vi "Potting Data from Inspect Modules.vi"() -> ()   [LabVIEW 2011]
uses:
  Procedure Classes/Potting Procedure/Type Definitions/Inspect Modules - Module.ctl
  Shared Components/Vec3d Class/Vec3d Class.lvclass
  Shared Components/Utils/Type Definitions/Multi-Fiducial Image.ctl
  Shared Components/Utils/Type Definitions/Physical Image.ctl
  <vilib>/vision/Image Controls.llb/IMAQ Image.ctl
  Shared Components/Utils/Type Definitions/Fiducial with Source.ctl
  Shared Components/Utils/Type Definitions/Fiducial Image.ctl
  Shared Components/SyringeTool Class/Type Definitions/Module Potting Data.ctl
  Shared Components/Utils/Type Definitions/3d Line.ctl
  Shared Components/Utils/Type Definitions/3d Point.ctl
panel:
  out "Module Potting Data":T1
  out "error out":errorcluster
  in  "error in":errorcluster
  in  "Module Data":T4={"TBM-TBM"={"Fiducial Image"={"Image Position"=refnum, "Image Reference"=refnum, "Field of View"={"x(mm)"=0.0, "y(mm)"=0.0}}, "Fiducials"=[]}, "TBM-HDI"={"Fiducial Image"={"Image Position"=refnum, "Image Reference"=refnum, "Field of View"={"x(mm)"=0.0, "y(mm)"=0.0}}, "Fiducials"=[]}, "Address Pads"={"Fiducial Image"={"Image Position"=refnum, "Image Reference"=refnum, "Field of View"={"x(mm)"=0.0, "y(mm)"=0.0}}, "Fiducials"=[]}, "HDI Bond Pad References"=[], "BBM Bond Pad References"=[], "HV-HDI"={"Fiducial Image"={"Image Position"=refnum, "Image Reference"=refnum, "Field of View"={"x(mm)"=0.0, "y(mm)"=0.0}}, "Selected Fiducial"={"Fiducial Image Coordinate"=refnum, "Fiducial Source"=enum."Pattern Recognition"}, "fiducial name"=""}, "HV-BBM"={"Fiducial Image"={"Image Position"=refnum, "Image Reference"=refnum, "Field of View"={"x(mm)"=0.0, "y(mm)"=0.0}}, "Selected Fiducial"={"Fiducial Image Coordinate"=refnum, "Fiducial Source"=enum."Pattern Recognition"}, "fiducial name"=""}, "Chuck"=0, "Slot"=0, "Potting Selection"={"HDI Bond Pads"=[TRUE, TRUE, TRUE, TRUE, TRUE, TRUE, TRUE, TRUE, TRUE, TRUE, TRUE, TRUE, TRUE, TRUE, TRUE, TRUE], "BBM Bond Pads"=[TRUE, TRUE, TRUE, TRUE, TRUE, TRUE, TRUE, TRUE, TRUE, TRUE, TRUE, TRUE, TRUE, TRUE, TRUE, TRUE], "TBM Inner"={"Top"=TRUE, "Left"=TRUE, "Bottom"=TRUE, "Right"=TRUE}, "TBM Outer"={"Top"=TRUE, "Left"=TRUE, "Bottom"=TRUE, "Right"=TRUE}, "Address Pads"={"Top"=TRUE, "Bottom"=TRUE}, "High Voltage"={"HDI"=TRUE, "BBM"=TRUE}}}
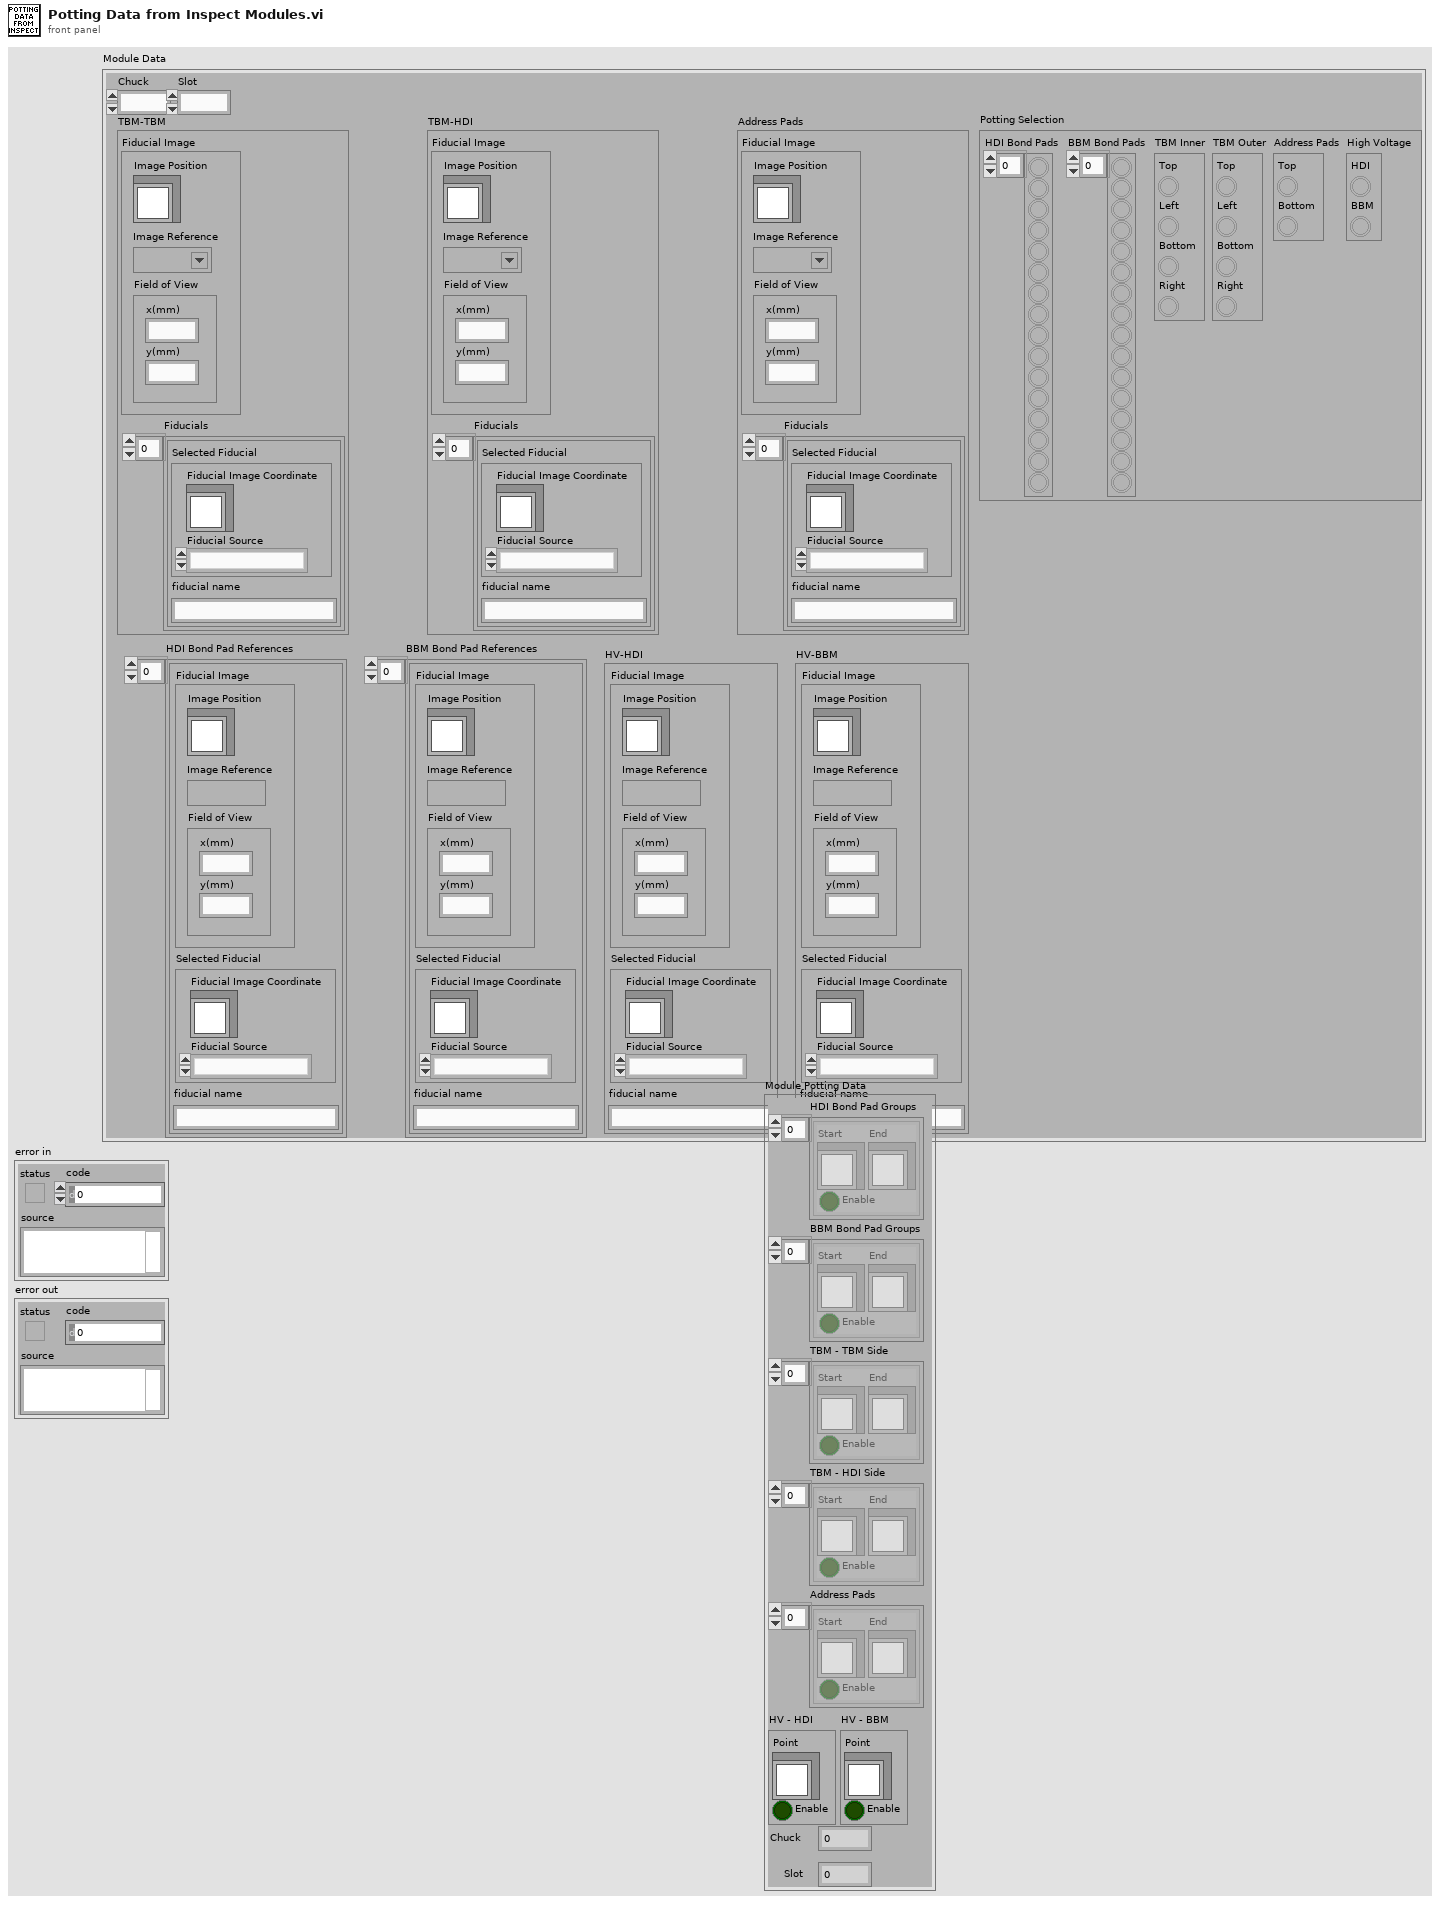
[diagram p1: front panel]
types:
  T1 = typedef "Module Potting Data.ctl" = cluster{"HDI Bond Pad Groups":T2[], "BBM Bond Pad Groups":T2[], "TBM - TBM Side":T2[], "TBM - HDI Side":T2[], "Address Pads":T2[], "Chuck":i32, "Slot":i32, "HV - HDI":T3, "HV - BBM":T3}
  T2 = typedef "3d Line.ctl" = cluster{"Start":refnum<class "Vec3d Class.lvclass">, "End":refnum<class "Vec3d Class.lvclass">, "Enable":bool}
  T3 = typedef "3d Point.ctl" = cluster{"Point":refnum<class "Vec3d Class.lvclass">, "Enable":bool}
  T4 = typedef "Inspect Modules - Module.ctl" = cluster{"TBM-TBM":T5, "TBM-HDI":T5, "Address Pads":T5, "HDI Bond Pad References":T9[], "BBM Bond Pad References":T9[], "HV-HDI":T9, "HV-BBM":T9, "Chuck":i32, "Slot":i32, "Potting Selection":cluster{"HDI Bond Pads":bool[], "BBM Bond Pads":bool[], "TBM Inner":cluster{"Top":bool, "Left":bool, "Bottom":bool, "Right":bool}, "TBM Outer":cluster{"Top":bool, "Left":bool, "Bottom":bool, "Right":bool}, "Address Pads":cluster{"Top":bool, "Bottom":bool}, "High Voltage":cluster{"HDI":bool, "BBM":bool}}}
  T5 = typedef "Multi-Fiducial Image.ctl" = cluster{"Fiducial Image":T6, "Fiducials":cluster{"Selected Fiducial":T8, "fiducial name":string}[]}
  T6 = typedef "Physical Image.ctl" = cluster{"Image Position":refnum<class "Vec3d Class.lvclass">, "Image Reference":T7, "Field of View":cluster{"x(mm)":dbl, "y(mm)":dbl}}
  T7 = typedef "IMAQ Image.ctl" = refnum<image>
  T8 = typedef "Fiducial with Source.ctl" = cluster{"Fiducial Image Coordinate":refnum<class "Vec3d Class.lvclass">, "Fiducial Source":enum16{"Pattern Recognition", "User", "Error", "Default"}}
  T9 = typedef "Fiducial Image.ctl" = cluster{"Fiducial Image":T6, "Selected Fiducial":T8, "fiducial name":string}
  T10 = cluster{"Top":bool, "Left":bool, "Bottom":bool, "Right":bool}
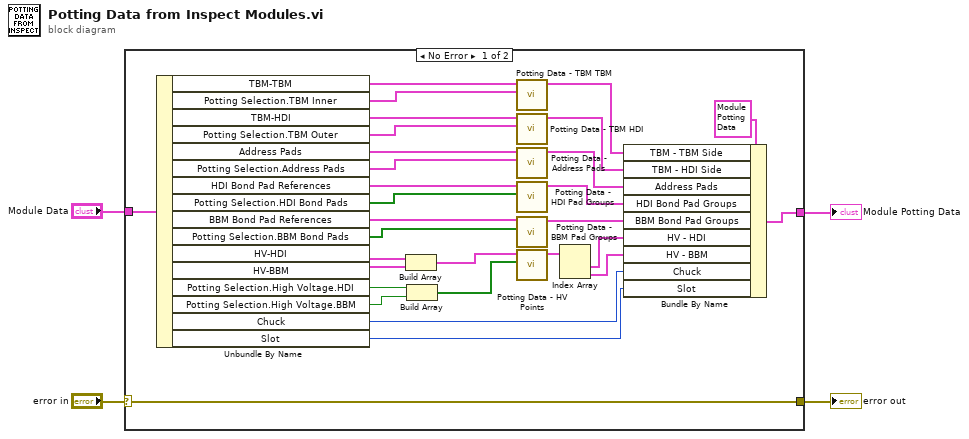
[diagram p0: block diagram]
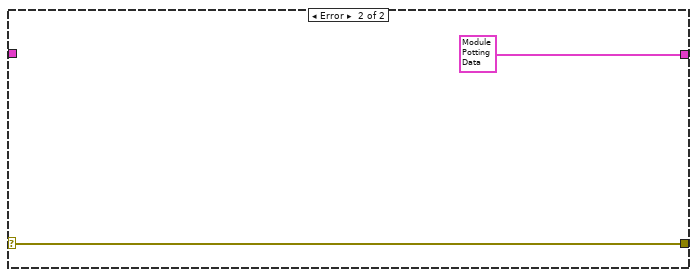
[diagram p2: hidden frame]
diagram:
  n1 = case shown="No Error" "error in" {
    selector: "error in" -> [w27 w36]
    tunnel: "Module Data" -> [w34 _]
    tunnel: [w27 w36] -> w2
    tunnel: [w8 T1 {"HDI Bond Pad Groups"=[], "BBM Bond Pad Groups"=[], "TBM - TBM Side"=[], "TBM - HDI Side"=[], "Address Pads"=[], "Chuck"=0, "Slot"=0, "HV - HDI"={"Point"=refnum, "Enable"=FALSE}, "HV - BBM"={"Point"=refnum, "Enable"=FALSE}} ("Module Potting Data")] -> w1
    frame No Error {
      n2 = Unbundle By Name(w34) -> ("TBM-TBM"=w33:T5, "Potting Selection.TBM Inner"=w32:T10, "TBM-HDI"=w31:T5, "Potting Selection.TBM Outer"=w30:T10, "Address Pads"=w29:T5, "Potting Selection.Address Pads"=w28:cluster{"Top":bool, "Bottom":bool}, "HDI Bond Pad References"=w26:T9[], "Potting Selection.HDI Bond Pads"=w25:bool[], "BBM Bond Pad References"=w24:T9[], "Potting Selection.BBM Bond Pads"=w23:bool[], "HV-HDI"=w22:T9, "HV-BBM"=w21:T9, "Potting Selection.High Voltage.HDI"=w20:bool, "Potting Selection.High Voltage.BBM"=w19:bool, "Chuck"=w10:i32, "Slot"=w9:i32)
      n3 = Build Array(w22, w21) -> (w17:T9[])
      n4 = Build Array(w20, w19) -> (w18:bool[])
      n5 = call "Potting Data - TBM TBM.vi"("TBM-TBM Selection"=w32, "TBM-TBM Data"=w33) -> ("Potting Lines"=w15:T2[])  [unwired: 9 in]
      n6 = call "Potting Data - TBM HDI.vi"("TBM-HDI Selection"=w30, "TBM-HDI Data"=w31) -> ("Potting Lines"=w14:T2[])  [unwired: 9 in]
      n7 = call "Potting Data - Address Pads.vi"("Address Pads Selection"=w28, "Address Pads Data"=w29) -> ("Potting Lines"=w13:T2[])  [unwired: 9 in]
      n8 = call "Potting Data - HDI Pad Groups.vi"("Potting Selection HDI Bond Pads"=w25, "HDI Bond Pad References"=w26) -> ("Potting Lines"=w12:T2[])  [unwired: 8 in, 1 out]
      n9 = call "Potting Data - BBM Pad Groups.vi"("Potting Selection BBM Bond Pads"=w23, "BBM Bond Pad References"=w24) -> ("Potting Lines"=w11:T2[])  [unwired: 8 in, 1 out]
      n10 = call "Potting Data - HV Points.vi"("HV Point Selection"=w18, "HV Point Data"=w17) -> ("HV Potting Points"=w7:T3[])  [unwired: 9 in]
      n11 = Index Array(array=w7) -> (element #1=w6:T3, element #2=w5:T3)  [unwired: 2 in]
      n12 = Bundle By Name(cluster=T1 {"HDI Bond Pad Groups"=[], "BBM Bond Pad Groups"=[], "TBM - TBM Side"=[], "TBM - HDI Side"=[], "Address Pads"=[], "Chuck"=0, "Slot"=0, "HV - HDI"={"Point"=refnum, "Enable"=FALSE}, "HV - BBM"={"Point"=refnum, "Enable"=FALSE}} ("Module Potting Data"), "TBM - TBM Side"=w15, "TBM - HDI Side"=w14, "Address Pads"=w13, "HDI Bond Pad Groups"=w12, "BBM Bond Pad Groups"=w11, "HV - HDI"=w6, "HV - BBM"=w5, "Chuck"=w10, "Slot"=w9) -> (w8:T1)
    }
    frame Error {
    }
  }
  "error out" <- w2
  "Module Potting Data" <- w1
